vi "Make Method Error Case.vi"(8 "error in (no error)":errorcluster, 11 "Error Checking Test in":refnum<class "Error Checking Test.lvclass">) -> (0 "error out":errorcluster, 3 "LUnit Test Case V2 out":refnum<class "LUnit Test Case.lvclass">)   [LabVIEW 2020, in "Error Checking Test.lvclass"]
uses:
  Error Checking Test.lvclass
  source/Core/LUnit Test Case/LUnit Test Case.lvclass
  source/Core/LUnit Test Case/LUnit Test Case.lvclass/LUnit Test Case.ctl
  <vilib>/Utility/LVClass/Get LV Class Name.vi
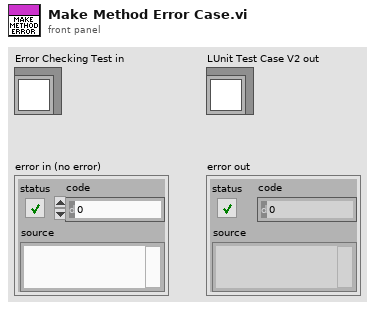
[diagram p1: front panel]
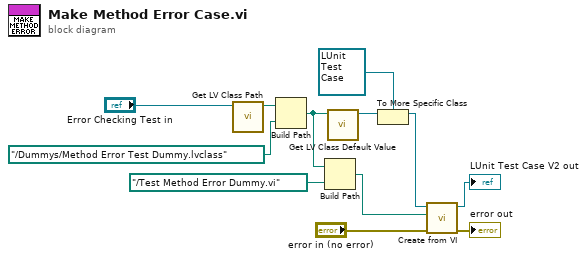
[diagram p0: block diagram]
diagram:
  n1 = call <vilib>:"Get LV Class Path.vi"("object"="Error Checking Test in") -> ("class path"=w7:path)  [unwired: 9 in, 1 out]
  n2 = Build Path(base path=w7, name or relative path=path "../Dummys/Method Error Test Dummy.lvclass") -> (appended path=w5:path)
  n3 = Build Path(base path=w5, name or relative path=path "../Test Method Error Dummy.vi") -> (appended path=w1:path)
  n4 = call <vilib>:"Get LV Class Default Value.vi"("class path"=w5) -> ("object"=w3:refnum<class>)  [unwired: 9 in, 1 out]
  n5 = To More Specific Class(target class=refnum<class "LUnit Test Case.lvclass"> refnum ("LUnit Test Case.lvclass"), reference=w3) -> (specific class reference=w2:refnum<class "LUnit Test Case.lvclass">)  [unwired: 1 in, 1 out]
  n6 = call "Create from VI.vi"("error in (no error)"="error in (no error)", "Test Method VI Path"=w1, "LUnit Test Case In"=w2) -> ("error out"=→"error out":errorcluster, "LUnit Test Case Out"=→"LUnit Test Case V2 out":refnum<class "LUnit Test Case.lvclass">)  [unwired: 7 in]
